vi "Configure FPGA.vi"(8 "error in":errorcluster, 11 "tCRD in":refnum<class "Open Path CRD.lvclass">) -> (0 "error out":errorcluster, 3 "tCRD out":refnum<class "Open Path CRD.lvclass">)   [LabVIEW 2015, in "Open Path CRD.lvclass"]
uses:
  Open Path CRD.lvclass
  FPGA/Rate.ctl
  Reusable/Session APIs/File Access/Config Data/Config Data.lvclass
  Reusable/Instrument/Instrument.lvclass/Instrument.ctl
  Reusable/Session APIs/File Access/Config Data/Config Data.lvclass/Config Data.ctl
  Open Path CRD.lvclass/Open Path CRD.ctl
  Reusable/CRDS/Main/CRDS.lvclass/CRDS.ctl
  Reusable/Instrument/Read Cfg Session.vi
  Reusable/Session APIs/File Access/Config Data/Accessors/Read Ref.vi
  Accessors/Write FPGA Ref.vi
  Reusable/CRDS/Main/Write NumCoadd.vi
  <vilib>/Utility/config.llb/Read Key (I32).vi
  <vilib>/FPGAPlugInAG/sbRIO-9637/niLvFpga_Open_sbRIO-9637.vi
  <vilib>/FPGAPlugInAG/sbRIO-9637/niLvFpga_Run_sbRIO-9637.vi
  <vilib>/Utility/error.llb/Error Cluster From Error Code.vi
  <vilib>/rvi/errors/niLvFpgaAdjustHostInterfaceError.vi
  <vilib>/rvi/interface/common/niFpgaWaitOnOcc.vi
  <userlib>/_Session Fwk/Session - Root.lvclass
  <vilib>/rvi/interface/nirviOpenFPGA/nirviOpenFPGA.xnode
  Open Path FPGA Ref.ctl
  FPGA Bitfiles/Handix_OpenPathCRD.lvbitx
  <vilib>/rvi/interface/nirviMethod/nirviMethod.xnode
  <vilib>/rvi/interface/nirviReadWriteControl/nirviReadWriteControl.xnode
  <vilib>/rvi/errors/niLvFpgaMergeErrorWithErrorCode.vi
  NiFpgaLv.dll
  <vilib>/Utility/config.llb/NI_LVConfig.lvlib
  <vilib>/FPGAPlugInAG/sbRIO-9637/niLvFpga_ConfigureFifo_sbRIO-9637.vi
  <vilib>/FPGAPlugInAG/sbRIO-9637/niLvFpga_StartFifo_sbRIO-9637.vi
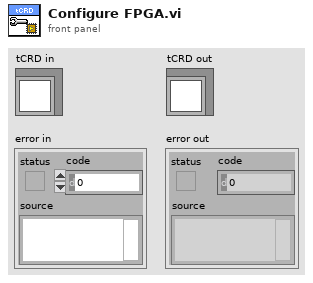
[diagram p1: front panel]
types:
  T1 = typedef "Rate.ctl" = u8
  T2 = typedef "Session - Root.lvclass/Session Handle.ctl" = refnum<data-value>
  T3 = typedef "NI_LVConfig.lvlib/Config Data RefNum.ctl" = refnum<k1>
  T4 = typedef "Open Path CRD.lvclass/Open Path FPGA Ref.ctl" = refnum<k20>
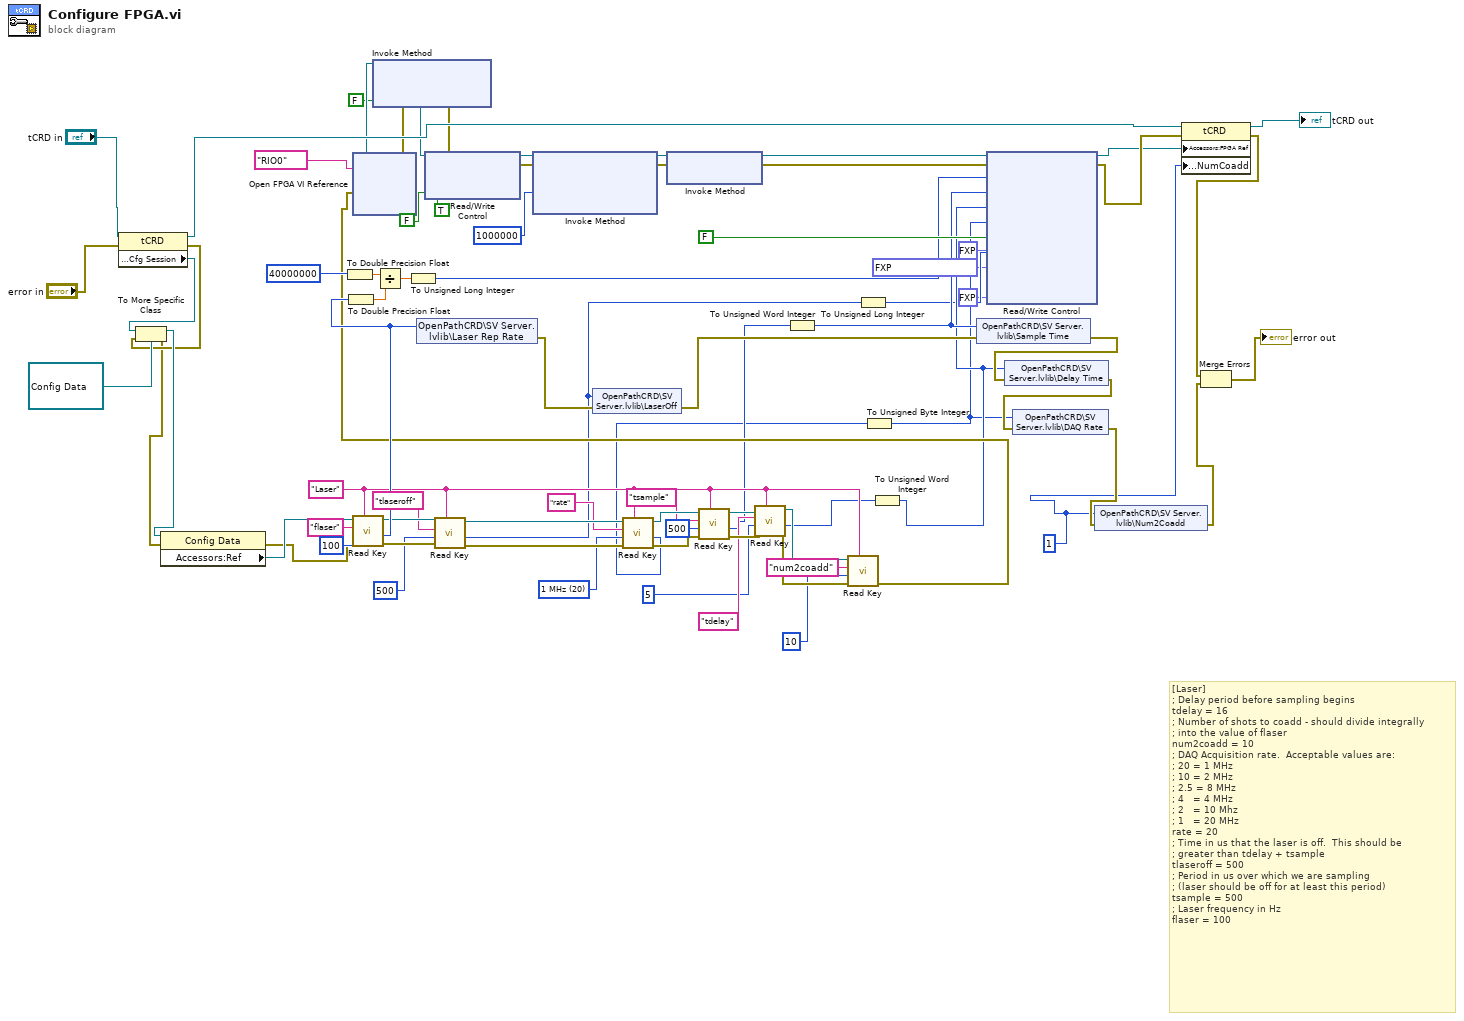
[diagram p0: block diagram]
diagram:
  w25 = 1 ("NumCoadd")
  w33 = "Laser" ("section")
  w45 = T1 20 items=["1 MHz"=20, "2 MHz"=10, "2.5 MHz"=8, "5 MHz"=4, "10 MHz"=2, "20MHz"=1] ("Rate")
  # "[Laser]\n; Delay period before sampling begins\ntdelay = 16\n; Number of shots to coadd - should divide integrally \n; into the value of flaser\nnum2coadd = 10\n; DAQ Acquisition rate.  Acceptable values are:\n; 20 = 1 MHz\n; 10 = 2 MHz\n; 2.5 = 8 MHz\n; 4   = 4 MHz\n; 2   = 10 Mhz\n; 1   = 20 MHz\nrate = 20\n; Time in us that the laser is off.  This should be\n; greater than tdelay + tsample\ntlaseroff = 500\n; Period in us over which we are sampling \n; (laser should be off for at least this period)\ntsample = 500\n; Laser frequency in Hz\nflaser = 100"
  n1 = property class="tCRD"(reference="tCRD in", error in="error in") -> (reference out=w11:refnum<class "Open Path CRD.lvclass">, error out=w13:errorcluster, "Accessors:Cfg Session"=w16:T2)
  n2 = To More Specific Class(target class=refnum<data-value> refnum, reference=w16, error in=w13) -> (specific class reference=w15:refnum<data-value>, error out=w9:errorcluster)
  n3 = property class="Config Data"(reference=w15, error in=w9) -> (error out=w31:errorcluster, "Accessors:Ref"=w56:T3)  [unwired: 1 out]
  n4 = To Double Precision Float(number=u32 40000000 ("Laser Rep Rate")) -> (double precision float=w73:dbl)
  n5 = call-poly <vilib>:"Read Key.vi"("section"=w33, "error in (no error)"=w31, "default value"=100, "key"="flaser", "refnum"=w56) -> ("error out"=w51:errorcluster, "value"=w54:i32, "refnum out"=w53:T3)  [unwired: 3 in, 1 out]
  n6 = To Double Precision Float(number=w54) -> (double precision float=w71:dbl)
  n7 = Divide(x=w73, y=w71) -> (x/y=w74:dbl)
  n8 = To Unsigned Long Integer(number=w74) -> (unsigned 32bit integer=w70:u32)
  n9 = shared-variable "OpenPathCRD\\SV Server.lvlib\\Laser Rep Rate"(w54) -> (error out=w64:errorcluster)  [unwired: 1 in]
  n10 = call-poly <vilib>:"Read Key.vi"("section"=w33, "error in (no error)"=w51, "default value"=u32 500 ("LaserOff"), "key"="tlaseroff", "refnum"=w53) -> ("error out"=w47:errorcluster, "value"=w20:i32, "refnum out"=w48:T3)  [unwired: 3 in, 1 out]
  n11 = shared-variable "OpenPathCRD\\SV Server.lvlib\\LaserOff"(w20, error in=w64) -> (error out=w63:errorcluster)
  n12 = call-poly <vilib>:"Read Key.vi"("section"=w33, "error in (no error)"=w47, "default value"=w45, "key"="rate", "refnum"=w48) -> ("error out"=w43:errorcluster, "value"=w18:i32, "refnum out"=w44:T3)  [unwired: 3 in, 1 out]
  n13 = call-poly <vilib>:"Read Key.vi"("section"=w33, "error in (no error)"=w43, "default value"=500, "key"="tsample", "refnum"=w44) -> ("error out"=w40:errorcluster, "value"=w24:i32, "refnum out"=w41:T3)  [unwired: 3 in, 1 out]
  n14 = call-poly <vilib>:"Read Key.vi"("section"=w33, "error in (no error)"=w40, "default value"=u16 5 ("Delay (us)"), "key"="tdelay", "refnum"=w41) -> ("error out"=w35:errorcluster, "value"=w22:i32, "refnum out"=w36:T3)  [unwired: 3 in, 1 out]
  n15 = To Unsigned Word Integer(number=w24) -> (unsigned 16bit integer=w23:u16)
  n16 = call-poly <vilib>:"Read Key.vi"("section"=w33, "error in (no error)"=w35, "default value"=u8 10 ("Num2Coadd"), "key"="num2coadd", "refnum"=w36) -> ("error out"=w30:errorcluster)  [unwired: 3 in, 3 out]
  n17 = xnode "Open FPGA VI Reference"("error in"=w30, "resource name"=tag "RIO0") -> ("FPGA VI Reference Out"=w7:T4, "error out"=w8:errorcluster)
  n18 = xnode "Invoke Method"("FPGA VI Reference In"=w7, "error in"=w8, "Wait Until Done (F)"=FALSE) -> ("FPGA VI Reference Out"=w6:T4, "error out"=w5:errorcluster)
  n19 = xnode ("Read/Write Control")("FPGA VI Reference In"=w6, "error in"=w5, "Pause Digitizer"=TRUE, "Reverse?"=FALSE) -> ("FPGA VI Reference Out"=w29:T4, "error out"=w28:errorcluster)
  n20 = xnode "Invoke Method"("FPGA VI Reference In"=w29, "error in"=w28, "Requested Depth"=u32 1000000) -> ("FPGA VI Reference Out"=w77:T4, "error out"=w76:errorcluster)  [unwired: 1 out]
  n21 = xnode "Invoke Method"("FPGA VI Reference In"=w77, "error in"=w76) -> ("FPGA VI Reference Out"=w27:T4, "error out"=w26:errorcluster)
  n22 = To Unsigned Long Integer(number=w20) -> (unsigned 32bit integer=w19:u32)
  n23 = To Unsigned Byte Integer(number=w18) -> (unsigned 8bit integer=w17:u8)
  n24 = To Unsigned Word Integer(number=w22) -> (unsigned 16bit integer=w21:u16)
  n25 = shared-variable "OpenPathCRD\\SV Server.lvlib\\Sample Time"(w23, error in=w63) -> (error out=w69:errorcluster)
  n26 = xnode "Read/Write Control"("FPGA VI Reference In"=w27, "error in"=w26, "Cylce (ticks)"=w70, "Sample Time (us)"=w23, "Delay (us)"=w21, "Rate"=w17, "Pause Digitizer"=FALSE, "LaserOff (us)"=w19, "p_slope"=fxp<+/-,16,1> 0.999969482421875, "p_offset"=fxp<+/-,16,1> 0.0, "u_slope"=fxp<+,9,9> 1.0) -> ("FPGA VI Reference Out"=w57:T4, "error out"=w60:errorcluster)
  n27 = shared-variable "OpenPathCRD\\SV Server.lvlib\\Delay Time"(w21, error in=w69) -> (error out=w68:errorcluster)
  n28 = shared-variable "OpenPathCRD\\SV Server.lvlib\\DAQ Rate"(w17, error in=w68) -> (error out=w65:errorcluster)
  n29 = shared-variable "OpenPathCRD\\SV Server.lvlib\\Num2Coadd"(w25, error in=w65) -> (error out=w62:errorcluster)
  n30 = property class="tCRD"(reference=w11, error in=w60, "Accessors:FPGA Ref"=w57, "Accessors:NumCoadd"=w25) -> (reference out=→"tCRD out":refnum<class "Open Path CRD.lvclass">, error out=w58:errorcluster)
  n31 = Merge Errors(w58, w62) -> (→"error out":errorcluster)
